vi "AutoRunDaily.vi"() -> ()   [LabVIEW 2012]
panel:
  out "date/time":string
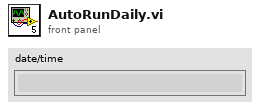
[diagram p1: front panel]
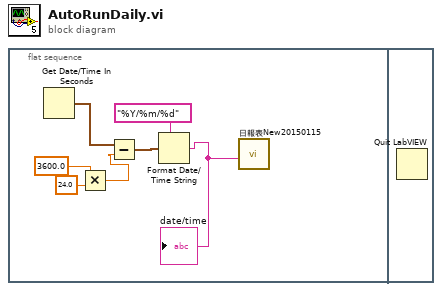
[diagram p0: block diagram]
diagram:
  n1 = flat-sequence {
    frame #0 {
      n2 = Get Date/Time In Seconds() -> (seconds since 1Jan1904=w7:timestamp)
      n3 = Multiply(x=3600.0, y=24.0) -> (x*y=w5:dbl)
      n4 = Subtract(x=w7, y=w5) -> (x-y=w4:timestamp)
      n5 = Format Date/Time String(time format string (%c)="%Y/%m/%d", seconds (now)=w4) -> (date/time string=w1:string)  [unwired: 1 in]
      "date/time" <- w1
      n6 = call "日報表New20150115.vi"("End Date"=w1) -> ()  [unwired: 10 in, 1 out]
    }
    frame #1 {
      n7 = Quit LabVIEW() -> ()  [unwired: 1 in]
    }
  }
